vi "Accessor_Read Ordered deps.vi"(8 "error in (no error)":errorcluster, 11 "SolutionBuilder in":refnum<class "SolutionBuilder.lvclass">) -> (0 "error out":errorcluster, 2 "Ordered deps":refnum<class "ProjectItem.lvclass">[](array[class]), 3 "SolutionBuilder out":refnum<class "SolutionBuilder.lvclass">)   [LabVIEW 2019, in "SolutionBuilder.lvlib" / "SolutionBuilder.lvclass"]
uses:
  SolutionBuilder.lvclass
  ProjectItem/ProjectItem.lvclass
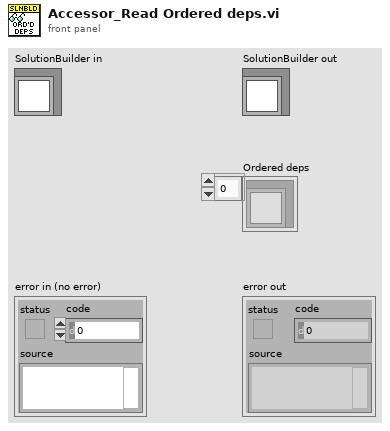
[diagram p1: front panel]
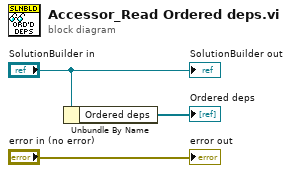
[diagram p0: block diagram]
diagram:
  n1 = Unbundle By Name("SolutionBuilder in") -> ("Ordered deps"=→"Ordered deps":refnum<class "ProjectItem.lvclass">[])
  "error out" <- "error in (no error)"
  "SolutionBuilder out" <- "SolutionBuilder in"
